vi "Write RT Variables.vi"(8 "error in (no error)":errorcluster, 10 "RT Variables.lvclass":refnum<class "RT Variables.lvclass">, 11 "functionbase in":refnum<class "functionbase.lvclass">) -> (0 "error out":errorcluster, 3 "functionbase out":refnum<class "functionbase.lvclass">)   [LabVIEW 2019, in "LSL.lvlib" / "functionbase.lvclass"]
uses:
  functionbase.lvclass
  variables/RT Variables/RT Variables.lvclass
  functionbase.lvclass/functionbase.ctl
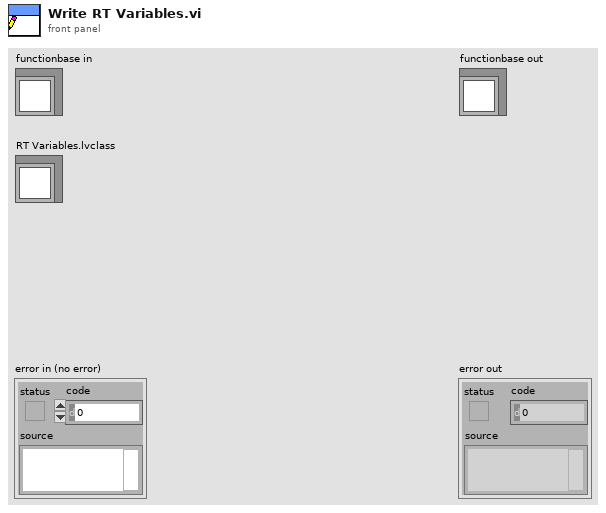
[diagram p1: front panel]
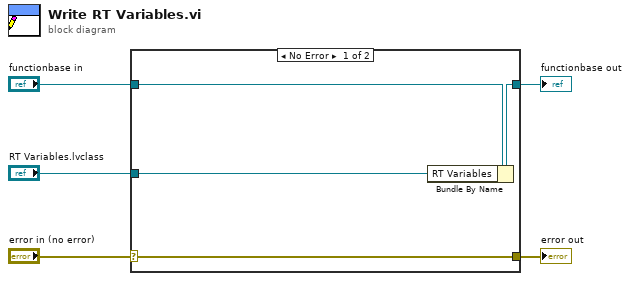
[diagram p0: block diagram]
diagram:
  n1 = case shown="No Error" "error in (no error)" {
    selector: "error in (no error)" -> [w9 w10]
    tunnel: [w9 w10] -> w4
    tunnel: [w7 w11] -> w2
    tunnel: "functionbase in" -> [w8 w11]
    tunnel: "RT Variables.lvclass" -> [w6 _]
    frame No Error {
      n2 = Bundle By Name(cluster=w8, "RT Variables"=w6) -> (w7:refnum<class "functionbase.lvclass">)
    }
    frame Error {
    }
  }
  "error out" <- w4
  "functionbase out" <- w2
